vi "PH_PSDBController.panel.vi"(0 "object ref":refnum<vi>, 5 "error in (no error)":errorcluster) -> (19 "error out":errorcluster)   [LabVIEW 2014, in "PH_PSDBController.lvlib"]
doc: "By this VI a hardware switch can be monitored and switched. \n\nThe indicators \"FALSE\", \"TRUE\" and \"SWITCH STATE\" show the value of the Beckhoff-Tag: blue indicates bad tag status reference problems, darkgreen false and lightgreen true. If everything is working fine, \"FALSE\" and \"SWITCH STATE\" should show the same value, while \"TRUE\" has the opposite value. The caption of the sensors for \"FALSE\" and \"TRUE\" are taken out of the database. In case of only one or no sensor these GUI elements are not shown at all.\n\nThe oval button switches. It should be in the same state as the \"SWITCH STATE\" indicator. \n\n\"Delete Instance\" disconnects and removes the instance from the PCS.\n\n\nLicense Agreement for this software:\n\nCopyright (C)\nGesellschaft für Schwerionenforschung, GSI\nPlanckstr. 1\n64291 Darmstadt\nGermany\n\nContact: D.Beck@gsi.de \n\nThis program is free software; you can redistribute it and/or modify it under the terms of the GNU General Public License as published by the Free Software Foundation; either version 2 of the license, or (at your option) any later version.\n\nThis program is distributed in the hope that it will be useful, but WITHOUT ANYW ARRANTY; without even the implied warranty of MERCHANTABILITY or FITNESS FOR A PARTICULAR PURPOSE. See the GNU General License for more details (http://www.gnu.org).\n\nGesellschaft für Schwerionenforschung, GSI\nPlanckstr. 1, 64291 Darmstadt, Germany\nFor all questions and ideas contact: M.Richter@gsi.de, H.Brand@gsi.de or D.Beck@gsi.de.\nLast update: 18-DEC-2002"
uses:
  PH_PSDBController.lvlib
  PH_PSDBWriter/PH_PSDBWriter.Data Status.ctl
  PH_StatusHandler/PH_StatusHandler.GUI element.ctl
  PH_PSDBWriter/PH_PSDBWriter.PHELIX-Subsystems.ctl
  CSCore/CSObj/CSObj.lvlib
  PH_Common/PH_Common.lvlib
  CSCore/CSSystem/CSSystemLib/CSSystemLib.lvlib
  PH_Class/PH_Class.lvlib
  PH_StatusHandler/PH_StatusHandler.lvlib
  PH_PSDBWriter/PH_PSDBWriter.lvlib
panel:
  out "Instances with Errors":string[](array[string])
  out "Sequencer SM State":string
  in  "Tab Control":T1(tab)
  out "Data Status BBs":cluster{"Instance":string, "Data Status":T2}[](array[cluster]) {"Data Status" items=["no info", "no Data collection", "no problem", "Error getting the ID", "Error writing Data", "Error getting the subsystem", "Error getting the Shot ID", "Error getting the Shot Types", "Error getting the Experiments", "Error verifying wanted Shottype", "Error verifying wanted Experiment"]}
  out "Data PPMA PUs":cluster{"Instance":string, "Data Status":T2}[](array[cluster]) {"Data Status" items=["no info", "no Data collection", "no problem", "Error getting the ID", "Error writing Data", "Error getting the subsystem", "Error getting the Shot ID", "Error getting the Shot Types", "Error getting the Experiments", "Error verifying wanted Shottype", "Error verifying wanted Experiment"]}
  out "Data PPPA PUs":cluster{"Instance":string, "Data Status":T2}[](array[cluster]) {"Data Status" items=["no info", "no Data collection", "no problem", "Error getting the ID", "Error writing Data", "Error getting the subsystem", "Error getting the Shot ID", "Error getting the Shot Types", "Error getting the Experiments", "Error verifying wanted Shottype", "Error verifying wanted Experiment"]}
  out "Data Cont 601 PUs":cluster{"Instance":string, "Data Status":T2}[](array[cluster]) {"Data Status" items=["no info", "no Data collection", "no problem", "Error getting the ID", "Error writing Data", "Error getting the subsystem", "Error getting the Shot ID", "Error getting the Shot Types", "Error getting the Experiments", "Error verifying wanted Shottype", "Error verifying wanted Experiment"]}
  out "Data Status Switches":cluster{"Instance":string, "Data Status":T2}[](array[cluster]) {"Data Status" items=["no info", "no Data collection", "no problem", "Error getting the ID", "Error writing Data", "Error getting the subsystem", "Error getting the Shot ID", "Error getting the Shot Types", "Error getting the Experiments", "Error verifying wanted Shottype", "Error verifying wanted Experiment"]}
  out "Data Status Powermeter":cluster{"Instance":string, "Data Status":T2}[](array[cluster]) {"Data Status" items=["no info", "no Data collection", "no problem", "Error getting the ID", "Error writing Data", "Error getting the subsystem", "Error getting the Shot ID", "Error getting the Shot Types", "Error getting the Experiments", "Error verifying wanted Shottype", "Error verifying wanted Experiment"]}
  out "Data M-Link":cluster{"Instance":string, "Data Status":T2}[](array[cluster]) {"Data Status" items=["no info", "no Data collection", "no problem", "Error getting the ID", "Error writing Data", "Error getting the subsystem", "Error getting the Shot ID", "Error getting the Shot Types", "Error getting the Experiments", "Error verifying wanted Shottype", "Error verifying wanted Experiment"]}
  out "Data Calorimeter":cluster{"Instance":string, "Data Status":T2}[](array[cluster]) {"Data Status" items=["no info", "no Data collection", "no problem", "Error getting the ID", "Error writing Data", "Error getting the subsystem", "Error getting the Shot ID", "Error getting the Shot Types", "Error getting the Experiments", "Error verifying wanted Shottype", "Error verifying wanted Experiment"]}
  out "Data Status O2 Monitor":cluster{"Instance":string, "Data Status":T2}[](array[cluster]) {"Data Status" items=["no info", "no Data collection", "no problem", "Error getting the ID", "Error writing Data", "Error getting the subsystem", "Error getting the Shot ID", "Error getting the Shot Types", "Error getting the Experiments", "Error verifying wanted Shottype", "Error verifying wanted Experiment"]}
  out "Data Status Mercury Monitor":cluster{"Instance":string, "Data Status":T2}[](array[cluster]) {"Data Status" items=["no info", "no Data collection", "no problem", "Error getting the ID", "Error writing Data", "Error getting the subsystem", "Error getting the Shot ID", "Error getting the Shot Types", "Error getting the Experiments", "Error verifying wanted Shottype", "Error verifying wanted Experiment"]}
  out "Data PA Chiller":cluster{"Instance":string, "Data Status":T2}[](array[cluster]) {"Data Status" items=["no info", "no Data collection", "no problem", "Error getting the ID", "Error writing Data", "Error getting the subsystem", "Error getting the Shot ID", "Error getting the Shot Types", "Error getting the Experiments", "Error verifying wanted Shottype", "Error verifying wanted Experiment"]}
  out "Data AWG 510":cluster{"Instance":string, "Data Status":T2}[](array[cluster]) {"Data Status" items=["no info", "no Data collection", "no problem", "Error getting the ID", "Error writing Data", "Error getting the subsystem", "Error getting the Shot ID", "Error getting the Shot Types", "Error getting the Experiments", "Error verifying wanted Shottype", "Error verifying wanted Experiment"]}
  out "Cams":cluster{"Instance":string, "Data Status":T2}[](array[cluster]) {"Data Status" items=["no info", "no Data collection", "no problem", "Error getting the ID", "Error writing Data", "Error getting the subsystem", "Error getting the Shot ID", "Error getting the Shot Types", "Error getting the Experiments", "Error verifying wanted Shottype", "Error verifying wanted Experiment"]}
  out "Data Hamamatsu Cams":cluster{"Instance":string, "Data Status":T2}[](array[cluster]) {"Data Status" items=["no info", "no Data collection", "no problem", "Error getting the ID", "Error writing Data", "Error getting the subsystem", "Error getting the Shot ID", "Error getting the Shot Types", "Error getting the Experiments", "Error verifying wanted Shottype", "Error verifying wanted Experiment"]}
  out "Image Operators":cluster{"Instance":string, "Data Status":T2}[](array[cluster]) {"Data Status" items=["no info", "no Data collection", "no problem", "Error getting the ID", "Error writing Data", "Error getting the subsystem", "Error getting the Shot ID", "Error getting the Shot Types", "Error getting the Experiments", "Error verifying wanted Shottype", "Error verifying wanted Experiment"]}
  out "OO Spectrometer":cluster{"Instance":string, "Data Status":T2}[](array[cluster]) {"Data Status" items=["no info", "no Data collection", "no problem", "Error getting the ID", "Error writing Data", "Error getting the subsystem", "Error getting the Shot ID", "Error getting the Shot Types", "Error getting the Experiments", "Error verifying wanted Shottype", "Error verifying wanted Experiment"]}
  out "Current Meas":cluster{"Instance":string, "Data Status":T2}[](array[cluster]) {"Data Status" items=["no info", "no Data collection", "no problem", "Error getting the ID", "Error writing Data", "Error getting the subsystem", "Error getting the Shot ID", "Error getting the Shot Types", "Error getting the Experiments", "Error verifying wanted Shottype", "Error verifying wanted Experiment"]}
  out "PP Conductivity Measurement":cluster{"Instance":string, "Data Status":T2}[](array[cluster]) {"Data Status" items=["no info", "no Data collection", "no problem", "Error getting the ID", "Error writing Data", "Error getting the subsystem", "Error getting the Shot ID", "Error getting the Shot Types", "Error getting the Experiments", "Error verifying wanted Shottype", "Error verifying wanted Experiment"]}
  out "TEK 7000":cluster{"Instance":string, "Data Status":T2}[](array[cluster]) {"Data Status" items=["no info", "no Data collection", "no problem", "Error getting the ID", "Error writing Data", "Error getting the subsystem", "Error getting the Shot ID", "Error getting the Shot Types", "Error getting the Experiments", "Error verifying wanted Shottype", "Error verifying wanted Experiment"]}
  out "Vacuum Controls":cluster{"Instance":string, "Data Status":T2}[](array[cluster]) {"Data Status" items=["no info", "no Data collection", "no problem", "Error getting the ID", "Error writing Data", "Error getting the subsystem", "Error getting the Shot ID", "Error getting the Shot Types", "Error getting the Experiments", "Error verifying wanted Shottype", "Error verifying wanted Experiment"]}
  out "BNCs":cluster{"Instance":string, "Data Status":T2}[](array[cluster]) {"Data Status" items=["no info", "no Data collection", "no problem", "Error getting the ID", "Error writing Data", "Error getting the subsystem", "Error getting the Shot ID", "Error getting the Shot Types", "Error getting the Experiments", "Error verifying wanted Shottype", "Error verifying wanted Experiment"]}
  out "SRDGs 535":cluster{"Instance":string, "Data Status":T2}[](array[cluster]) {"Data Status" items=["no info", "no Data collection", "no problem", "Error getting the ID", "Error writing Data", "Error getting the subsystem", "Error getting the Shot ID", "Error getting the Shot Types", "Error getting the Experiments", "Error verifying wanted Shottype", "Error verifying wanted Experiment"]}
  out "SRDGs 645":cluster{"Instance":string, "Data Status":T2}[](array[cluster]) {"Data Status" items=["no info", "no Data collection", "no problem", "Error getting the ID", "Error writing Data", "Error getting the subsystem", "Error getting the Shot ID", "Error getting the Shot Types", "Error getting the Experiments", "Error verifying wanted Shottype", "Error verifying wanted Experiment"]}
  out "Sixpacks":cluster{"Instance":string, "Data Status":T2}[](array[cluster]) {"Data Status" items=["no info", "no Data collection", "no problem", "Error getting the ID", "Error writing Data", "Error getting the subsystem", "Error getting the Shot ID", "Error getting the Shot Types", "Error getting the Experiments", "Error verifying wanted Shottype", "Error verifying wanted Experiment"]}
  out "Data Beckhoff Motion":cluster{"Instance":string, "Data Status":T2}[](array[cluster]) {"Data Status" items=["no info", "no Data collection", "no problem", "Error getting the ID", "Error writing Data", "Error getting the subsystem", "Error getting the Shot ID", "Error getting the Shot Types", "Error getting the Experiments", "Error verifying wanted Shottype", "Error verifying wanted Experiment"]}
  out "Data SHS Analysis":cluster{"Instance":string, "Data Status":T2}[](array[cluster]) {"Data Status" items=["no info", "no Data collection", "no problem", "Error getting the ID", "Error writing Data", "Error getting the subsystem", "Error getting the Shot ID", "Error getting the Shot Types", "Error getting the Experiments", "Error verifying wanted Shottype", "Error verifying wanted Experiment"]}
  out "Data Status 6P Waveplates":cluster{"Instance":string, "Data Status":T2}[](array[cluster]) {"Data Status" items=["no info", "no Data collection", "no problem", "Error getting the ID", "Error writing Data", "Error getting the subsystem", "Error getting the Shot ID", "Error getting the Shot Types", "Error getting the Experiments", "Error verifying wanted Shottype", "Error verifying wanted Experiment"]}
  out "Data Status 6P Switch":cluster{"Instance":string, "Data Status":T2}[](array[cluster]) {"Data Status" items=["no info", "no Data collection", "no problem", "Error getting the ID", "Error writing Data", "Error getting the subsystem", "Error getting the Shot ID", "Error getting the Shot Types", "Error getting the Experiments", "Error verifying wanted Shottype", "Error verifying wanted Experiment"]}
  out "Data Status 6P GUI":cluster{"Instance":string, "Data Status":T2}[](array[cluster]) {"Data Status" items=["no info", "no Data collection", "no problem", "Error getting the ID", "Error writing Data", "Error getting the subsystem", "Error getting the Shot ID", "Error getting the Shot Types", "Error getting the Experiments", "Error verifying wanted Shottype", "Error verifying wanted Experiment"]}
  out "Data Revolver":cluster{"Instance":string, "Data Status":T2}[](array[cluster]) {"Data Status" items=["no info", "no Data collection", "no problem", "Error getting the ID", "Error writing Data", "Error getting the subsystem", "Error getting the Shot ID", "Error getting the Shot Types", "Error getting the Experiments", "Error verifying wanted Shottype", "Error verifying wanted Experiment"]}
  out "Data Status SSAC":cluster{"Instance":string, "Data Status":T2}[](array[cluster]) {"Data Status" items=["no info", "no Data collection", "no problem", "Error getting the ID", "Error writing Data", "Error getting the subsystem", "Error getting the Shot ID", "Error getting the Shot Types", "Error getting the Experiments", "Error verifying wanted Shottype", "Error verifying wanted Experiment"]}
  out "Data Status Sequencer":cluster{"Instance":string, "Data Status":T2}[](array[cluster]) {"Data Status" items=["no info", "no Data collection", "no problem", "Error getting the ID", "Error writing Data", "Error getting the subsystem", "Error getting the Shot ID", "Error getting the Shot Types", "Error getting the Experiments", "Error verifying wanted Shottype", "Error verifying wanted Experiment"]}
  out "Data 4 Pos Selector":cluster{"Instance":string, "Data Status":T2}[](array[cluster]) {"Data Status" items=["no info", "no Data collection", "no problem", "Error getting the ID", "Error writing Data", "Error getting the subsystem", "Error getting the Shot ID", "Error getting the Shot Types", "Error getting the Experiments", "Error verifying wanted Shottype", "Error verifying wanted Experiment"]}
  in  "Take Snapshot":bool caption="Force Timing"
  in  "Get PSDB Info":bool caption="Force Timing"
  out "Experiment Description":string
  in  "Shottype":i16(ring)=3 items=["experiment shot"=1, "test shot"=2, "snapshot"=3, "other"=4]
  in  "Experiment":i16(ring) items=["P1"=1]
  in  "Shot Comment":string
  out "active Subsystems":T3 caption="PHELIX Subsysteme" items=["Miscellaneous", "fs-Frontend", "ns-Frontend", "PreAmp", "MainAmp", "MAS", "COS", "Beamline", "Experiment Laserbay", "Experiment Laserlabor", "Experiment Z6", "Timing", "Pulsed Power"]
  out "Controller Data Status":T2 items=["no info", "no Data collection", "no problem", "Error getting the ID", "Error writing Data", "Error getting the subsystem", "Error getting the Shot ID", "Error getting the Shot Types", "Error getting the Experiments", "Error verifying wanted Shottype", "Error verifying wanted Experiment"]
  out "Status":T4 caption="Enabling State"
  out "Current Shot ID":i32
  in  "Exit":bool
  in  "Delete":bool
  # "PCS"
  # "3.40"
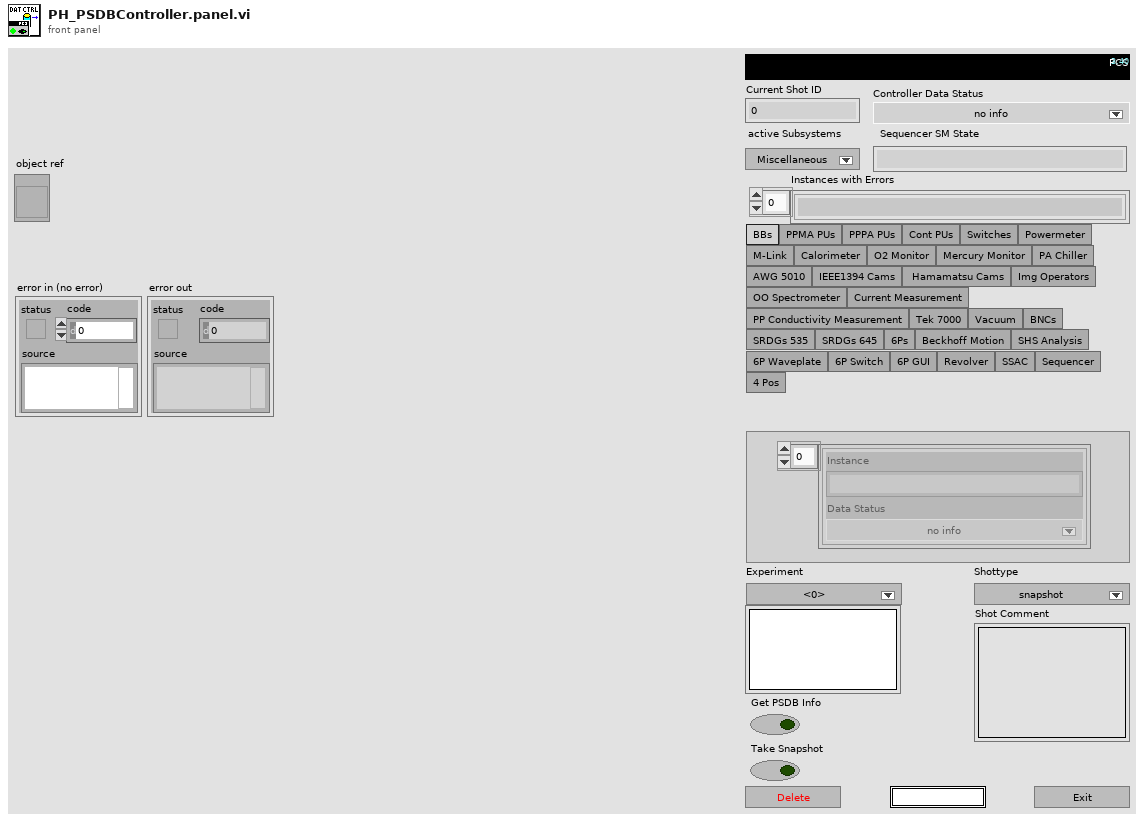
[diagram p1: front panel]
types:
  T1 = enum32{"BBs", "PPMA PUs", "PPPA PUs", "Cont PUs", "Switches", "Powermeter", "M-Link", "Calorimeter", "O2 Monitor", "Mercury Monitor", "PA Chiller", "AWG 5010", "IEEE1394 Cams", " Hamamatsu Cams", "Img Operators", "OO Spectrometer", "Current Measurement", "PP Conductivity Measurement", "Tek 7000", "Vacuum", "BNCs", "SRDGs 535", "SRDGs 645", "6Ps", "Beckhoff Motion", "SHS Analysis", "6P Waveplate", "6P Switch", "6P GUI", "Revolver", "SSAC", "Sequencer", "4 Pos"}
  T2 = typedef "PH_PSDBWriter.lvlib/PH_PSDBWriter.Data Status.ctl" = i16
  T3 = typedef "PH_PSDBWriter.lvlib/PH_PSDBWriter.PHELIX-Subsystems.ctl" = i32
  T4 = typedef "PH_StatusHandler.lvlib/PH_StatusHandler.GUI element.ctl" = u16
  T5 = typedef "PH_PSDBController.lvlib/PH_PSDBController.i attribute.ctl" = cluster{"GUI Refs":cluster{"Data Status":refnum<vi>, "Current Shot ID":refnum<vi>, "active Subsystems":refnum<vi>, "Experiment Description":refnum<vi>, "Shot Comment":refnum<vi>, "Experiment":refnum<vi>, "Shottype":refnum<vi>, "Sequencer SM State":refnum<vi>, "Instances with Errors":refnum<vi>}, "Service ID Shot ID":i32, "Service ID wanted Subsystem":i32, "Data Status":T2, "Shotinformation":cluster{"Current Experiment ID":i32, "Current Shot Type":i32, "Current Comment":string}, "Data taking?":bool, "Service ID current Shottype":i32, "Service ID current Experiment":i32, "Service ID currentShot Comment":i32, "Service ID possible Shottypes":i32, "Service ID possible Experiments":i32, "possible Experiments":T6[], "possible Shottypes":T6[], "List":cluster{"Info":cluster{"Instance":string, "Data Status":T2}[], "GUI Ref":refnum<vi>, "Classname":string}[], "Subsystems Off?":cluster{"PHELIX_Beamline_fs_YLF_BL_Status":bool, "PHELIX_Beamline_ns_BL_Status":bool, "PHELIX_Beamline_PA_Input_BL_Status":bool, "PHELIX_Beamline_PA_MA_BL_Status":bool, "PHELIX_Beamline_MA_Z6_BL_Status":bool, "PHELIX_Beamline_MA_LB_BL_Status":bool, "PHELIX_Beamline_PA_LL_BL_Status":bool}, "PSDB Credentials":T7}
  T6 = typedef "PSDB.lvlib/PSDB_Info.ctl" = cluster{"Name":string, "Description":string, "ID":i32}
  T7 = typedef "PH_Common.lvlib/PH_Connection.PSDB Credentials.ctl" = cluster{"PW":string, "ID":string, "DS":string}
  T8 = cluster{"Info":cluster{"Instance":string, "Data Status":T2}[], "GUI Ref":refnum<vi>, "Classname":string}[]
  T9 = cluster{"Info":cluster{"Instance":string, "Data Status":T2}[], "GUI Ref":refnum<vi>, "Classname":string}
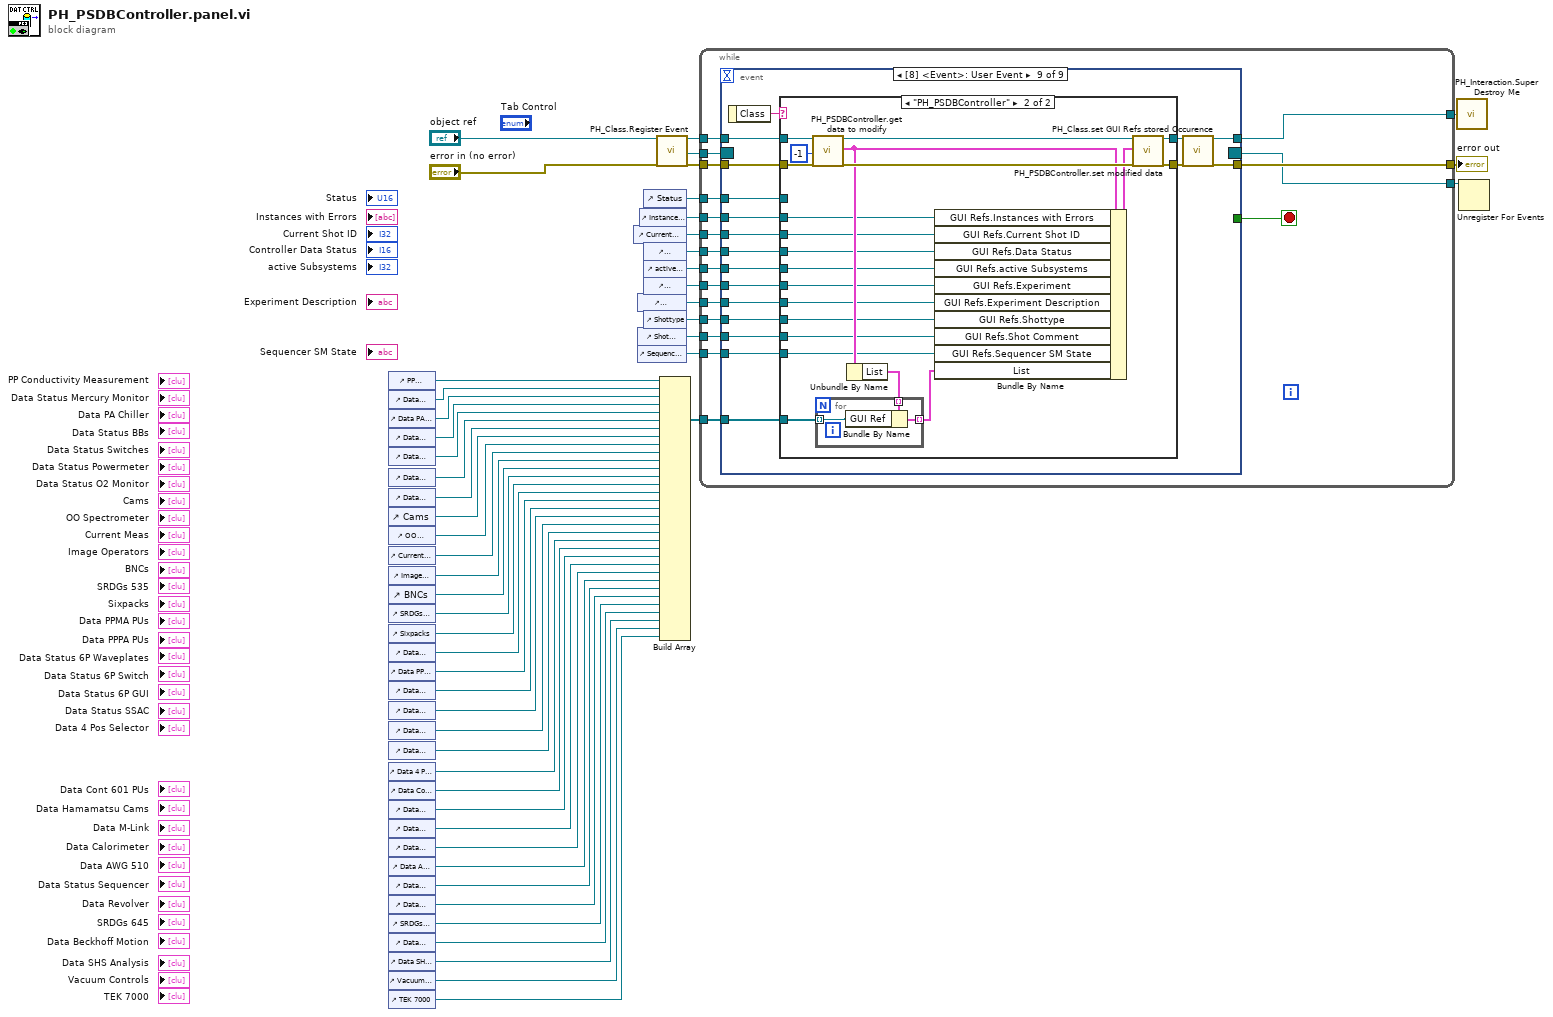
[diagram p0: block diagram]
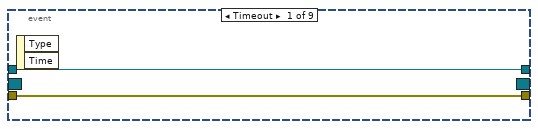
[diagram p2: hidden frame]
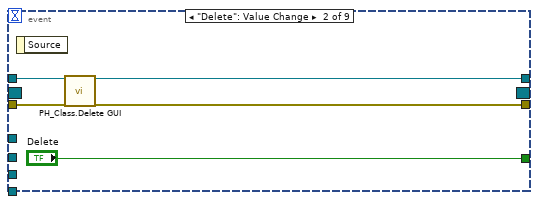
[diagram p3: hidden frame]
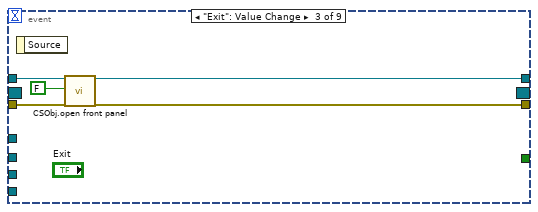
[diagram p4: hidden frame]
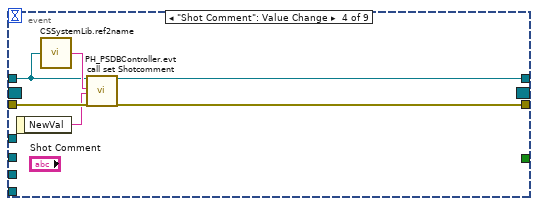
[diagram p5: hidden frame]
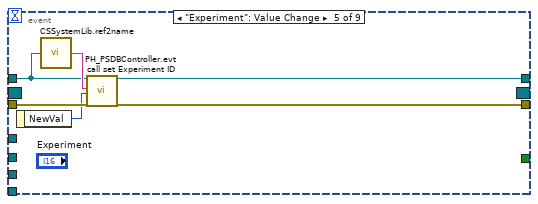
[diagram p6: hidden frame]
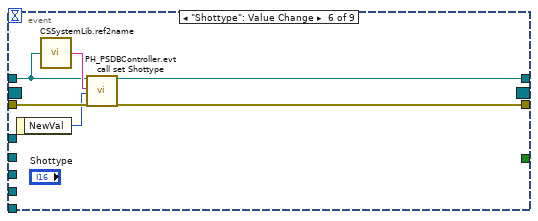
[diagram p7: hidden frame]
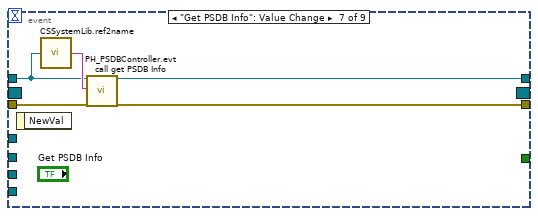
[diagram p8: hidden frame]
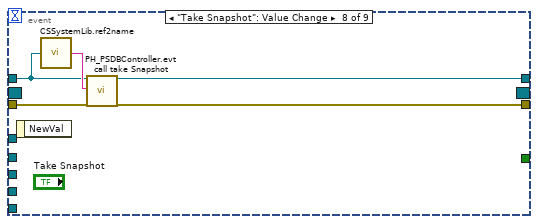
[diagram p9: hidden frame]
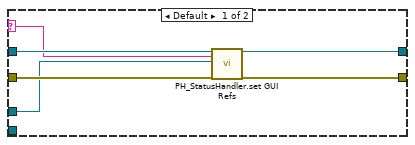
[diagram p10: hidden frame]
diagram:
  n1 = control-ref of="PP Conductivity Measurement"() -> (w32:refnum<vi>)
  n2 = control-ref of="Data Status Mercury Monitor"() -> (w31:refnum<vi>)
  n3 = control-ref of="Data PA Chiller"() -> (w30:refnum<vi>)
  n4 = control-ref of="Data Status BBs"() -> (w50:refnum<vi>)
  n5 = control-ref of="Data Status Switches"() -> (w49:refnum<vi>)
  n6 = control-ref of="Data Status Powermeter"() -> (w48:refnum<vi>)
  n7 = control-ref of="Data Status O2 Monitor"() -> (w47:refnum<vi>)
  n8 = control-ref of="Cams"() -> (w46:refnum<vi>)
  n9 = control-ref of="OO Spectrometer"() -> (w45:refnum<vi>)
  n10 = control-ref of="Current Meas"() -> (w44:refnum<vi>)
  n11 = control-ref of="Image Operators"() -> (w43:refnum<vi>)
  n12 = control-ref of="BNCs"() -> (w42:refnum<vi>)
  n13 = control-ref of="SRDGs 535"() -> (w41:refnum<vi>)
  n14 = control-ref of="Sixpacks"() -> (w40:refnum<vi>)
  n15 = control-ref of="Data PPMA PUs"() -> (w39:refnum<vi>)
  n16 = control-ref of="Data PPPA PUs"() -> (w38:refnum<vi>)
  n17 = control-ref of="Data Status 6P Waveplates"() -> (w37:refnum<vi>)
  n18 = control-ref of="Data Status 6P Switch"() -> (w36:refnum<vi>)
  n19 = control-ref of="Data Status 6P GUI"() -> (w35:refnum<vi>)
  n20 = control-ref of="Data Status SSAC"() -> (w34:refnum<vi>)
  n21 = control-ref of="Data 4 Pos Selector"() -> (w33:refnum<vi>)
  n22 = control-ref of="Data Cont 601 PUs"() -> (w13:refnum<vi>)
  n23 = control-ref of="Data Hamamatsu Cams"() -> (w12:refnum<vi>)
  n24 = control-ref of="Data M-Link"() -> (w11:refnum<vi>)
  n25 = control-ref of="Data Calorimeter"() -> (w10:refnum<vi>)
  n26 = control-ref of="Data AWG 510"() -> (w9:refnum<vi>)
  n27 = control-ref of="Data Status Sequencer"() -> (w8:refnum<vi>)
  n28 = control-ref of="Data Revolver"() -> (w7:refnum<vi>)
  n29 = control-ref of="SRDGs 645"() -> (w6:refnum<vi>)
  n30 = control-ref of="Data Beckhoff Motion"() -> (w5:refnum<vi>)
  n31 = control-ref of="Data SHS Analysis"() -> (w4:refnum<vi>)
  n32 = control-ref of="Vacuum Controls"() -> (w3:refnum<vi>)
  n33 = control-ref of="TEK 7000"() -> (w2:refnum<vi>)
  n34 = control-ref of="Current Shot ID"() -> (w23:refnum<vi>)
  n35 = control-ref of="Experiment Description"() -> (w19:refnum<vi>)
  n36 = control-ref of="Shot Comment"() -> (w17:refnum<vi>)
  n37 = control-ref of="Sequencer SM State"() -> (w16:refnum<vi>)
  n38 = control-ref of="Instances with Errors"() -> (w24:refnum<vi>)
  n39 = control-ref of="Status"() -> (w1:refnum<vi>)
  n40 = control-ref of="Controller Data Status"() -> (w22:refnum<vi>)
  n41 = control-ref of="active Subsystems"() -> (w21:refnum<vi>)
  n42 = control-ref of="Experiment"() -> (w20:refnum<vi>)
  n43 = control-ref of="Shottype"() -> (w18:refnum<vi>)
  n44 = call "PH_Class.Register Event.vi"("i ref in"="object ref", "error in (no error)"="error in (no error)") -> ("i ref out"=w29:refnum<vi>, "Event Registration Refnum"=w27:refnum<event-registration>, "error out"=w28:errorcluster)  [unwired: 15 in]
  n45 = Build Array(w32, w31, w30, w50, w49, w48, w47, w46, w45, w44, w43, w42, w41, w40, w39, w38, w37, w36, w35, w34, w33, w13, w12, w11, w10, w9, w8, w7, w6, w5, w4, w3, w2) -> (w25:refnum<vi>[])
  n46 = while {
    tunnel: w29 -> [w68]
    tunnel: [w67] -> w51
    tunnel: w28 -> [w70]
    tunnel: [w69] -> w52
    tunnel: w27 -> [w65]
    tunnel: [w64] -> w26
    tunnel: w25 -> [w63]
    tunnel: w24 -> [w62]
    tunnel: w1 -> [w61]
    tunnel: w23 -> [w60]
    tunnel: w22 -> [w59]
    tunnel: w21 -> [w58]
    tunnel: w20 -> [w57]
    tunnel: w19 -> [w56]
    tunnel: w18 -> [w55]
    tunnel: w17 -> [w54]
    tunnel: w16 -> [w53]
    stop <- w66 stop-if-true
    n47 = event shown="[8] <Event>: User Event" {
      selector: w65 -> [_ _ _ _ _ _ _ _ _]
      dyn-events: [_ _ _ _ _ _ _ _ _] -> w64
      timeout: _ -> [_ _ _ _ _ _ _ _ _]
      tunnel: w68 -> [w71 w73 w81 w84 w90 w96 w101 w106 w128]
      tunnel: w70 -> [w72 w77 w80 w88 w94 w100 w105 w110 w127]
      tunnel: [w72 w76 w79 w87 w93 w99 w104 w109 w123] -> w69
      tunnel: [w71 w75 w78 w86 w92 w98 w103 w108 w124] -> w67
      tunnel: [_ "Delete" _ _ _ _ _ _ _] -> w66
      tunnel: w63 -> [_ _ _ _ _ _ _ _ w121]
      tunnel: w62 -> [_ _ _ _ _ _ _ _ w120]
      tunnel: w61 -> [_ _ _ _ _ _ _ _ w119]
      tunnel: w60 -> [_ _ _ _ _ _ _ _ w118]
      tunnel: w59 -> [_ _ _ _ _ _ _ _ w117]
      tunnel: w58 -> [_ _ _ _ _ _ _ _ w116]
      tunnel: w57 -> [_ _ _ _ _ _ _ _ w115]
      tunnel: w56 -> [_ _ _ _ _ _ _ _ w114]
      tunnel: w55 -> [_ _ _ _ _ _ _ _ w113]
      tunnel: w54 -> [_ _ _ _ _ _ _ _ w112]
      tunnel: w53 -> [_ _ _ _ _ _ _ _ w111]
      event Timeout {
        n48 = event-data() -> ()  [unwired: 1 in, 2 out]
      }
      event "Delete": Value Change {
        n49 = event-data() -> ()  [unwired: 1 in, 1 out]
        n50 = call "PH_Class.Delete GUI.vi"("VI in"=w73, "error in (no error)"=w77) -> ("VI out"=w75:refnum<vi>, "error out"=w76:errorcluster)  [unwired: 16 in]
      }
      event "Exit": Value Change {
        n51 = event-data() -> ()  [unwired: 1 in, 1 out]
        n52 = call "CSObj.open front panel.vi"("i ref in"=w81, "frontPanelOpen"=FALSE ("front panel open"), "error in (no error)"=w80) -> ("i ref out"=w78:refnum<vi>, "error out"=w79:errorcluster)  [unwired: 15 in]
      }
      event "Shot Comment": Value Change {
        n53 = event-data() -> ("NewVal"=w83:string)  [unwired: 1 in]
        n54 = call "CSSystemLib.ref2name.vi"("obj refnum"=w84) -> ("name"=w85:string)
        n55 = call "PH_PSDBController.evt call set Shotcomment.vi"("i ref in"=w84, "Instance"=w85, "Shot Comment"=w83, "error in (no error)"=w88) -> ("i ref out"=w86:refnum<vi>, "error out"=w87:errorcluster)  [unwired: 14 in]
      }
      event "Experiment": Value Change {
        n56 = event-data() -> ("NewVal"=w89:i16)  [unwired: 1 in]
        n57 = call "CSSystemLib.ref2name.vi"("obj refnum"=w90) -> ("name"=w91:string)
        n58 = call "PH_PSDBController.evt call set Experiment ID.vi"("i ref in"=w90, "Instance"=w91, "Experiment"=w89, "error in (no error)"=w94) -> ("i ref out"=w92:refnum<vi>, "error out"=w93:errorcluster)  [unwired: 14 in]
      }
      event "Shottype": Value Change {
        n59 = event-data() -> ("NewVal"=w95:i16)  [unwired: 1 in]
        n60 = call "CSSystemLib.ref2name.vi"("obj refnum"=w96) -> ("name"=w97:string)
        n61 = call "PH_PSDBController.evt call set Shottype.vi"("i ref in"=w96, "Instance"=w97, "Shot Type"=w95, "error in (no error)"=w100) -> ("i ref out"=w98:refnum<vi>, "error out"=w99:errorcluster)  [unwired: 14 in]
      }
      event "Get PSDB Info": Value Change {
        n62 = event-data() -> ()  [unwired: 1 in, 1 out]
        n63 = call "CSSystemLib.ref2name.vi"("obj refnum"=w101) -> ("name"=w102:string)
        n64 = call "PH_PSDBController.evt call get PSDB Info.vi"("i ref in"=w101, "Instance"=w102, "error in (no error)"=w105) -> ("i ref out"=w103:refnum<vi>, "error out"=w104:errorcluster)  [unwired: 15 in]
      }
      event "Take Snapshot": Value Change {
        n65 = event-data() -> ()  [unwired: 1 in, 1 out]
        n66 = call "CSSystemLib.ref2name.vi"("obj refnum"=w106) -> ("name"=w107:string)
        n67 = call "PH_PSDBController.evt call take Snapshot.vi"("i ref in"=w106, "Instance"=w107, "error in (no error)"=w110) -> ("i ref out"=w108:refnum<vi>, "error out"=w109:errorcluster)  [unwired: 15 in]
      }
      event User Event {
        n68 = event-data() -> ("Class"=w122:string)  [unwired: 1 in]
        n69 = case shown="\"PH_PSDBController\"" w122 {
          selector: w122 -> [w130 _]
          tunnel: w128 -> [w132 w148]
          tunnel: w127 -> [w134 w147]
          tunnel: [w131 w146] -> w126
          tunnel: [w133 w145] -> w125
          tunnel: w121 -> [_ w144]
          tunnel: w120 -> [_ w143]
          tunnel: w119 -> [w129 _]
          tunnel: w118 -> [_ w142]
          tunnel: w117 -> [_ w141]
          tunnel: w116 -> [_ w140]
          tunnel: w115 -> [_ w139]
          tunnel: w114 -> [_ w138]
          tunnel: w113 -> [_ w137]
          tunnel: w112 -> [_ w136]
          tunnel: w111 -> [_ w135]
          frame Default {
            n70 = call "PH_StatusHandler.set GUI Refs.vi"("i ref in"=w132, "Class"=w130, "GUI Ref"=w129, "error in (no error)"=w134) -> ("i ref out"=w131:refnum<vi>, "error out"=w133:errorcluster)  [unwired: 14 in]
          }
          frame "PH_PSDBController" {
            n71 = call "PH_PSDBController.get data to modify.vi"("i ref in"=w148, "ms timeout (10000)"=-1, "error in (no error)"=w147) -> ("i ref out"=w153:refnum<vi>, "i attribute"=w150:T5, "error out"=w155:errorcluster)  [unwired: 13 in, 1 out]
            n72 = Unbundle By Name(w150) -> ("List"=w149:T8)
            n73 = for {
              tunnel: [w158] -> w151 mode=indexing
              tunnel: w144 -> [w157] mode=indexing
              tunnel: w149 -> [w156] mode=indexing
              n74 = Bundle By Name(cluster=w156, "GUI Ref"=w157) -> (w158:T9)
            }
            n75 = Bundle By Name(cluster=w150, "GUI Refs.Instances with Errors"=w143, "GUI Refs.Current Shot ID"=w142, "GUI Refs.Data Status"=w141, "GUI Refs.active Subsystems"=w140, "GUI Refs.Experiment"=w139, "GUI Refs.Experiment Description"=w138, "GUI Refs.Shottype"=w137, "GUI Refs.Shot Comment"=w136, "GUI Refs.Sequencer SM State"=w135, "List"=w151) -> (w152:T5)
            n76 = call "PH_PSDBController.set modified data.vi"("i ref in"=w153, "i attribute"=w152, "error in (no error)"=w155) -> ("i ref out"=w146:refnum<vi>, "error out"=w145:errorcluster)  [unwired: 15 in]
          }
        }
        n77 = call "PH_Class.set GUI Refs stored Occurence.vi"("i ref in"=w126, "error in (no error)"=w125) -> ("i ref out"=w124:refnum<vi>, "error out"=w123:errorcluster)  [unwired: 16 in]
      }
    }
  }
  "error out" <- w52
  n78 = call "PH_Interaction.Super Destroy Me.vi"("i ref out"=w51) -> ()
  n79 = Unregister For Events(event registration refnum=w26) -> ()  [unwired: 1 in, 1 out]
